vi "UpdateTimeout.vi"(7 "ReadOnlyIn":T1={"Qref"={"ValveCTR"=refnum, "Error"=refnum}, "UI_EN"=FALSE, "UserEventREF"={"TimeBasedProducer"={"Reg"=refnum, "Ref"=refnum}, "TimeBasedTempRead"={"Reg"=refnum, "Ref"=refnum}}, "UI_REF"=variant, "Paths"={"Log_Dir"=path "", "TempLog"=path "", "WateringLog"=path "", "Error"=path "", "Settings_Dir"=path "", "CFG.ini"=path "", "Plant_Digital_OP"=path "", "TimeTable"=path "", "Consol_Dir"=path "", "Input"=path "", "Output"=path "", "Timeout"=path "", "TimeoutTable"=path "", "Ch_Stat"=path "", "Temp"=path ""}, "PI_REF"={"IO"=enum."Remote", "Interface"=enum."Serial", "LINX Device Config"={"Interface"=enum."Serial", "COM Port"="COM13", "TCP Configuration"={"IP Address"="", "Port"=0}, "Device Family"=1, "Device ID"=1, "Device Name"="myRIO-1900", "TCP Ref"=refnum, "Channels"={"DI"=[0, 1, 2, 3, 4, 5, 6, 7, 8, 9, 10, 11, 12, 13, 14, 15, 16, 17, 18, 19, 20, 21, 22, 23, 24, 25, 26, 27, 28, 29, 30, 31, 32, 33, 34, 35, 36, 37, 38, 39, 40, 41, 42, 43, 44, 45, 46], "DO"=[0, 1, 2, 3, 4, 5, 6, 7, 8, 9, 10, 11, 12, 13, 14, 15, 16, 17, 18, 19, 20, 21, 22, 23, 24, 25, 26, 27, 28, 29, 30, 31, 32, 33, 34, 35, 36, 37, 38, 39, 40, 41, 42, 43, 44, 45, 46], "AI"=[0, 1, 2, 3, 4, 5, 6, 7, 8, 9, 10, 11], "AO"=[], "PWM"=[3, 5, 6, 9, 10], "QE"=[], "UART"=[0, 1], "I2C 2"=[0], "SPI"=[0], "CAN"=[], "Servo"=[], "AI Ref (V)"=0.0, "AI Resolution (Bits)"=0, "AO Ref (V)"=0.0, "AO Resolution (Bits)"=0}}}, "CFG"={"ProducerEn_PC"=FALSE, "Producer_PC_ms"=0, "ProducerEn_PI"=FALSE, "Producer_PI_ms"=0, "TempLogInterval"=15, "SystemResetTime"=0.0}} {"CFG"."SystemResetTime" format="%<%H:%M:%S>t"}, 8 "Error In":errorcluster, 11 "Read_WriteIN":T9={"Time Table"=[{"Set Time"=0.0, "Control"=enum."Time", "Duration[S]"=3.0, "Liter"=0.0, "Plant Name."="", "Watered"=FALSE, "Su"=FALSE, "Mo"=FALSE, "Tu"=FALSE, "We"=FALSE, "Th"=FALSE, "Fr"=FALSE, "Sa"=FALSE}, {"Set Time"=0.0, "Control"=enum."Time", "Duration[S]"=5.0, "Liter"=0.0, "Plant Name."="", "Watered"=FALSE, "Su"=FALSE, "Mo"=FALSE, "Tu"=FALSE, "We"=FALSE, "Th"=FALSE, "Fr"=FALSE, "Sa"=FALSE}, {"Set Time"=0.0, "Control"=enum."Time", "Duration[S]"=5.0, "Liter"=0.0, "Plant Name."="", "Watered"=FALSE, "Su"=FALSE, "Mo"=FALSE, "Tu"=FALSE, "We"=FALSE, "Th"=FALSE, "Fr"=FALSE, "Sa"=FALSE}], "Plants_Digital_OP"=[], "delta_ms_w_Index"={"delta_ms"=[], "Index"=[], "RunArray"=[]}, "TimeOutInfo"={"Timeout"=0, "ValveCTR"={"State"=enum."Open Valve", "Channel No"=0, "Duration[S]"=0.0}, "Index"=0}, "LoopName"=""} {"TimeOutInfo"."ValveCTR"."Channel No" items=["7"=7, "11"=11, "12"=12, "13"=13, "15"=15, "16"=16, "18"=18, "29"=29, "32"=32, "33"=33, "35"=35, "36"=36, "37"=37, "38"=38, "40"=40]; "delta_ms_w_Index"."RunArray"."Channel No" items=["7"=7, "11"=11, "12"=12, "13"=13, "15"=15, "16"=16, "18"=18, "29"=29, "32"=32, "33"=33, "35"=35, "36"=36, "37"=37, "38"=38, "40"=40]; "Plants_Digital_OP"."Channel No" items=["7"=7, "11"=11, "12"=12, "13"=13, "15"=15, "16"=16, "18"=18, "29"=29, "32"=32, "33"=33, "35"=35, "36"=36, "37"=37, "38"=38, "40"=40]; "Time Table"."Liter" min=0.0; "Time Table"."Set Time" format="%<%H:%M:%S>t"; "Time Table"."Duration[S]" min=0.0}) -> (0 "Error Out":errorcluster, 3 "Read_WriteOUT":T9={"Time Table"=[{"Set Time"=0.0, "Control"=enum."Time", "Duration[S]"=3.0, "Liter"=0.0, "Plant Name."="", "Watered"=FALSE, "Su"=FALSE, "Mo"=FALSE, "Tu"=FALSE, "We"=FALSE, "Th"=FALSE, "Fr"=FALSE, "Sa"=FALSE}, {"Set Time"=0.0, "Control"=enum."Time", "Duration[S]"=5.0, "Liter"=0.0, "Plant Name."="", "Watered"=FALSE, "Su"=FALSE, "Mo"=FALSE, "Tu"=FALSE, "We"=FALSE, "Th"=FALSE, "Fr"=FALSE, "Sa"=FALSE}, {"Set Time"=0.0, "Control"=enum."Time", "Duration[S]"=5.0, "Liter"=0.0, "Plant Name."="", "Watered"=FALSE, "Su"=FALSE, "Mo"=FALSE, "Tu"=FALSE, "We"=FALSE, "Th"=FALSE, "Fr"=FALSE, "Sa"=FALSE}], "Plants_Digital_OP"=[], "delta_ms_w_Index"={"delta_ms"=[], "Index"=[], "RunArray"=[]}, "TimeOutInfo"={"Timeout"=0, "ValveCTR"={"State"=enum."Open Valve", "Channel No"=0, "Duration[S]"=0.0}, "Index"=0}, "LoopName"=""} {"TimeOutInfo"."ValveCTR"."Channel No" items=["7"=7, "11"=11, "12"=12, "13"=13, "15"=15, "16"=16, "18"=18, "29"=29, "32"=32, "33"=33, "35"=35, "36"=36, "37"=37, "38"=38, "40"=40]; "delta_ms_w_Index"."RunArray"."Channel No" items=["7"=7, "11"=11, "12"=12, "13"=13, "15"=15, "16"=16, "18"=18, "29"=29, "32"=32, "33"=33, "35"=35, "36"=36, "37"=37, "38"=38, "40"=40]; "Plants_Digital_OP"."Channel No" items=["7"=7, "11"=11, "12"=12, "13"=13, "15"=15, "16"=16, "18"=18, "29"=29, "32"=32, "33"=33, "35"=35, "36"=36, "37"=37, "38"=38, "40"=40]; "Time Table"."Liter" min=0.0; "Time Table"."Set Time" format="%<%H:%M:%S>t"; "Time Table"."Duration[S]" min=0.0})   [LabVIEW 2020, in "TimeBasedProd.lvlib"]
uses:
  TimeBasedProd.lvlib
  TypeDef/Read_Write.ctl
  TimeTable/TypeDef/Time_Table.ctl
  TimeTable/TypeDef/Time_Table_CTR.ctl
  Digital_OP/TypeDef/Plant_OP_Map.ctl
  Digital_OP/TypeDef/Plant_OP_Map_CTR.ctl
  ValveCTRL/TypeDef/CHs_List.ctl
  TypeDef/TimeOutInfo.ctl
  ValveCTRL/TypeDef/Queue_Cluster.ctl
  ValveCTRL/TypeDef/States_Enum.ctl
  TypeDef/UpdateTimeOutinfo.ctl
  Main/TypeDef/ReadOnly.ctl
  Main/TypeDef/EventData.ctl
  <vilib>/MakerHub/LINX/Private/Type Defs/LINX Ref.ctl
  <vilib>/MakerHub/LINX/Private/Type Defs/Platform.ctl
  <vilib>/MakerHub/LINX/Private/Type Defs/Interface.ctl
  <vilib>/MakerHub/LINX/Private/Device/Type Defs/LINX Device Config.ctl
  <vilib>/MakerHub/LINX/Private/Device/Type Defs/TCP Config.ctl
  <vilib>/MakerHub/LINX/Private/Device/Type Defs/Channels.ctl
  Main/Init/ReadInitCFG/TypeDef/CFG_Cluster.ctl
  Time/Time.lvlib
  ValveCTRL/ValveCTRL.lvlib
  Main/Main.lvlib
  <vilib>/MakerHub/LINX/LMH-LINX.lvlib
  <vilib>/MakerHub/LINX/Private/Device/Device.lvlib
panel:
  # "Watering Days"
  # "Watering Days"
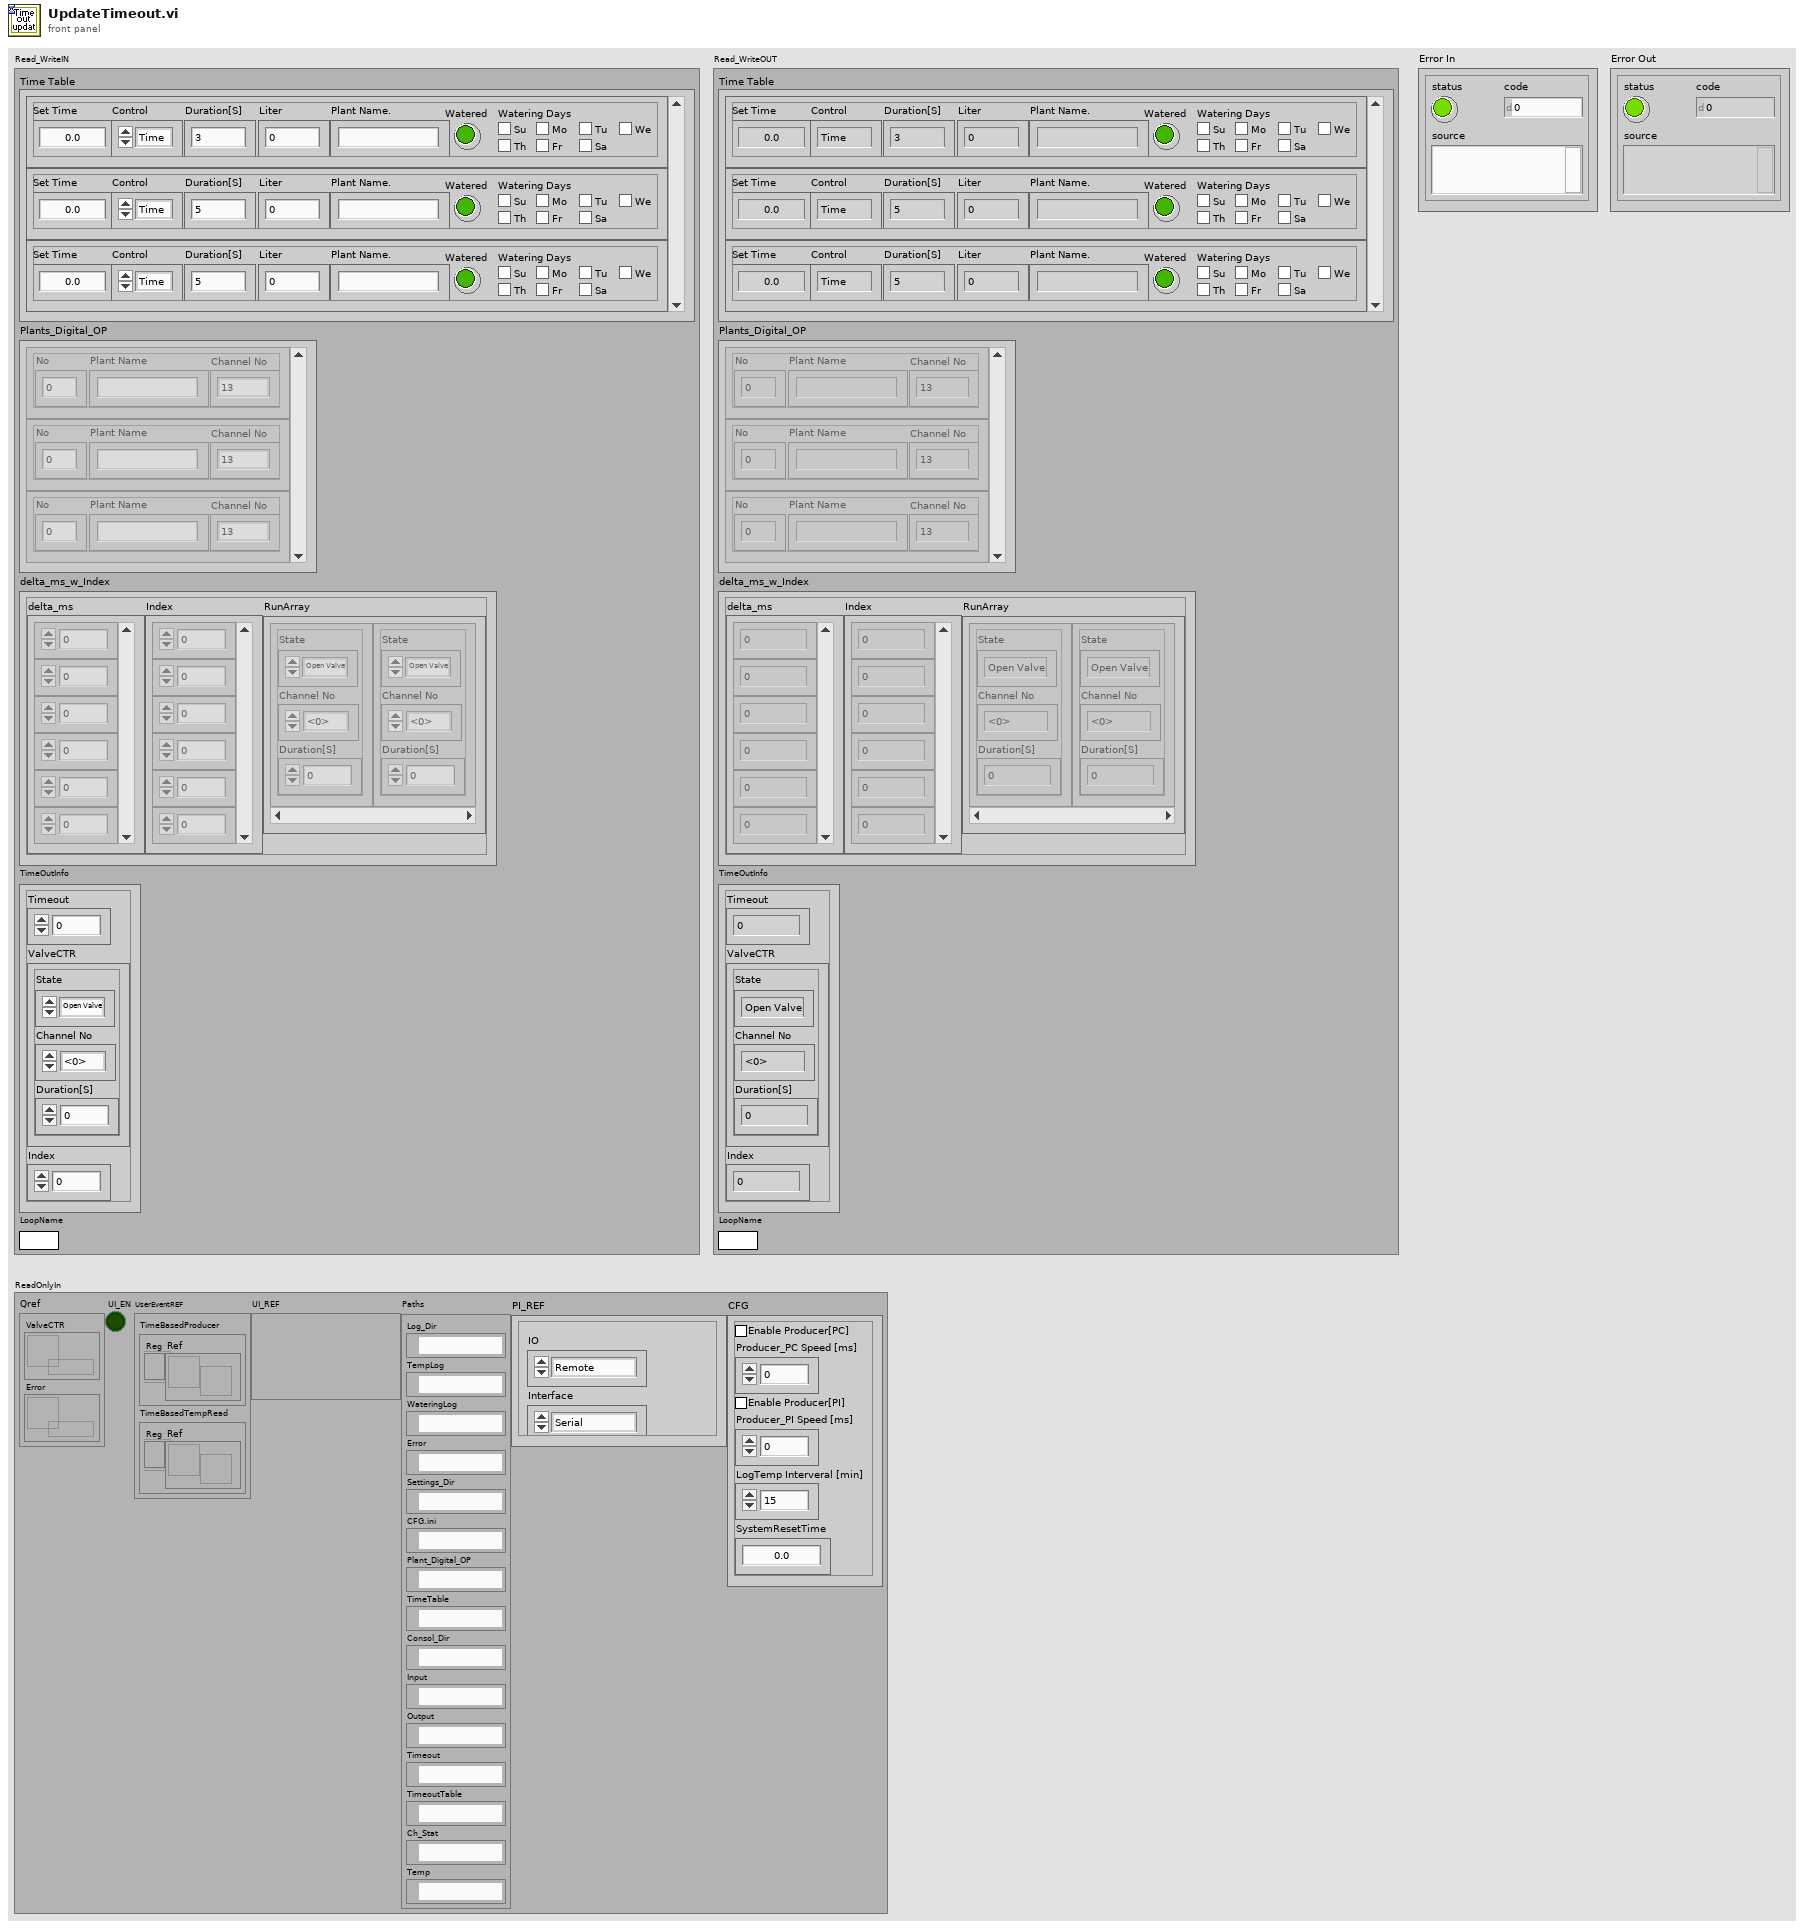
[diagram p1: front panel]
types:
  T1 = typedef "Main.lvlib/ReadOnly.ctl" = cluster{"Qref":cluster{"ValveCTR":refnum<queue>, "Error":refnum<queue>}, "UI_EN":bool, "UserEventREF":cluster{"TimeBasedProducer":cluster{"Reg":refnum<event-registration>, "Ref":refnum<user-event>}, "TimeBasedTempRead":cluster{"Reg":refnum<event-registration>, "Ref":refnum<user-event>}}, "UI_REF":variant, "Paths":cluster{"Log_Dir":path, "TempLog":path, "WateringLog":path, "Error":path, "Settings_Dir":path, "CFG.ini":path, "Plant_Digital_OP":path, "TimeTable":path, "Consol_Dir":path, "Input":path, "Output":path, "Timeout":path, "TimeoutTable":path, "Ch_Stat":path, "Temp":path}, "PI_REF":T2, "CFG":T8}
  T2 = typedef "LMH-LINX.lvlib/LINX Ref.ctl" = cluster{"IO":T3, "Interface":T4, "LINX Device Config":T5}
  T3 = typedef "LMH-LINX.lvlib/Platform.ctl" = enum16{"Remote", "Local"}
  T4 = typedef "LMH-LINX.lvlib/Interface.ctl" = enum16{"Serial", "TCP"}
  T5 = typedef "LMH-LINX.lvlib/Device.lvlib/LINX Device Config.ctl" = cluster{"Interface":T4, "COM Port":refnum<visa-resource-name>, "TCP Configuration":T6, "Device Family":u8, "Device ID":u8, "Device Name":string, "TCP Ref":refnum<k5>, "Channels":T7}
  T6 = typedef "LMH-LINX.lvlib/Device.lvlib/TCP Config.ctl" = cluster{"IP Address":string, "Port":u16}
  T7 = typedef "LMH-LINX.lvlib/Channels.ctl" = cluster{"DI":u8[], "DO":u8[], "AI":u8[], "AO":u8[], "PWM":u8[], "QE":u8[], "UART":u8[], "I2C 2":u8[], "SPI":u8[], "CAN":u8[], "Servo":u8[], "AI Ref (V)":dbl, "AI Resolution (Bits)":u8, "AO Ref (V)":dbl, "AO Resolution (Bits)":u8}
  T8 = typedef "Main.lvlib/CFG_Cluster.ctl" = cluster{"ProducerEn_PC":bool, "Producer_PC_ms":u32, "ProducerEn_PI":bool, "Producer_PI_ms":u32, "TempLogInterval":u32, "SystemResetTime":dbl}
  T9 = typedef "TimeBasedProd.lvlib/Read_Write.ctl" = cluster{"Time Table":T10, "Plants_Digital_OP":T12, "delta_ms_w_Index":T15, "TimeOutInfo":T18, "LoopName":string}
  T10 = typedef "TimeBasedProd.lvlib/Time_Table.ctl" = T11[]
  T11 = typedef "TimeBasedProd.lvlib/Time_Table_CTR.ctl" = cluster{"Set Time":dbl, "Control":enum16{"Time", "Flow"}, "Duration[S]":dbl, "Liter":dbl, "Plant Name.":string, "Watered":bool, "Su":bool, "Mo":bool, "Tu":bool, "We":bool, "Th":bool, "Fr":bool, "Sa":bool}
  T12 = typedef "TimeBasedProd.lvlib/Plant_OP_Map.ctl" = T13[]
  T13 = typedef "TimeBasedProd.lvlib/Plant_OP_Map_CTR.ctl" = cluster{"No":u8, "Plant Name":string, "Channel No":T14}
  T14 = typedef "ValveCTRL.lvlib/CHs_List.ctl" = u8
  T15 = typedef "TimeBasedProd.lvlib/TimeOutInfo.ctl" = cluster{"delta_ms":i32[], "Index":i32[], "RunArray":T16[]}
  T16 = typedef "ValveCTRL.lvlib/Queue_Cluster.ctl" = cluster{"State":T17, "Channel No":T14, "Duration[S]":dbl}
  T17 = typedef "ValveCTRL.lvlib/States_Enum.ctl" = enum16{"Open Pump", "Open Valve", "Wait Valve", "Close Pump", "Close Valve", "Save State", "StopLoop", "ValidCh"}
  T18 = typedef "TimeBasedProd.lvlib/UpdateTimeOutinfo.ctl" = cluster{"Timeout":i32, "ValveCTR":T16, "Index":i32}
  T19 = enum16{"open", "replace", "create", "open or create", "replace or create", "replace or create with confirmation"}
  T20 = typedef "Time.lvlib/Local_DateTime_String.ctl" = cluster{"Local Date Time":string, "Local Date":string, "Local Time":string}
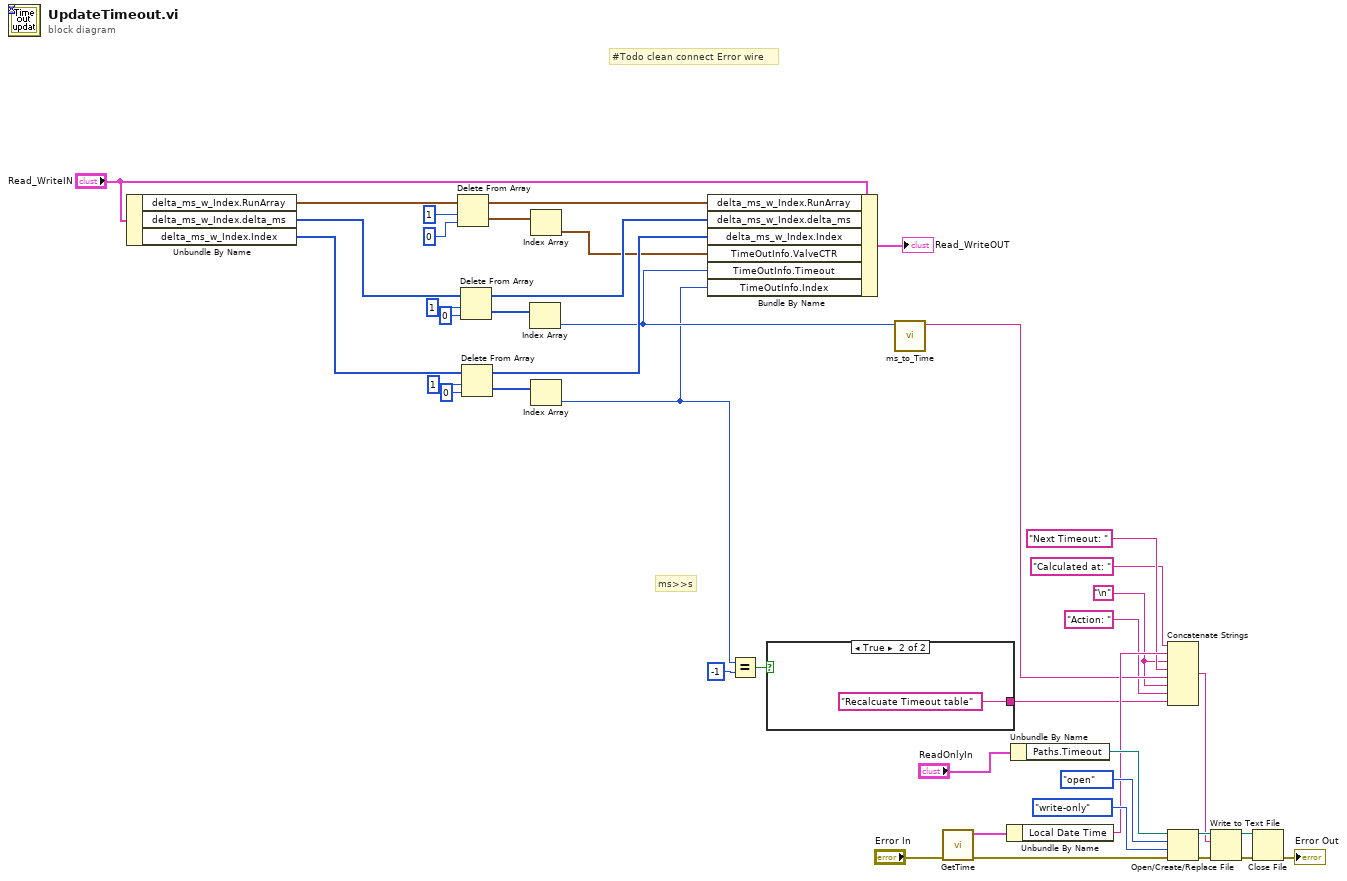
[diagram p0: block diagram]
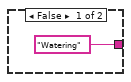
[diagram p2: hidden frame]
diagram:
  w3 = "\n"
  # "ms>>s"
  # "#Todo clean connect Error wire"
  n1 = Unbundle By Name("Read_WriteIN") -> ("delta_ms_w_Index.RunArray"=w33:T16[], "delta_ms_w_Index.delta_ms"=w41:i32[], "delta_ms_w_Index.Index"=w29:i32[])
  n2 = Delete From Array(array=w33, length=1, index=0) -> (deleted portion=w40:T16[], array with subset deleted=w34:T16[])
  n3 = Delete From Array(array=w41, length=1, index=0) -> (deleted portion=w37:i32[], array with subset deleted=w42:i32[])
  n4 = Delete From Array(array=w29, length=1, index=0) -> (deleted portion=w32:i32[], array with subset deleted=w28:i32[])
  n5 = Index Array(array=w37) -> (element=w8:i32)  [unwired: 1 in]
  n6 = Index Array(array=w40) -> (element=w26:T16)  [unwired: 1 in]
  n7 = Index Array(array=w32) -> (element=w6:i32)  [unwired: 1 in]
  n8 = Bundle By Name(cluster="Read_WriteIN", "delta_ms_w_Index.RunArray"=w34, "delta_ms_w_Index.delta_ms"=w42, "delta_ms_w_Index.Index"=w28, "TimeOutInfo.ValveCTR"=w26, "TimeOutInfo.Timeout"=w8, "TimeOutInfo.Index"=w6) -> (→"Read_WriteOUT":T9)
  n9 = Equal?(x=w6, y=-1) -> (x = y?=w4:bool)
  n10 = case shown="True" w4 {
    tunnel: ["Watering" ("string") "Recalcuate Timeout table" ("string")] -> w1
    frame False {
    }
    frame True {
    }
  }
  n11 = call "ms_to_Time.vi"("TimeOut[ms]"=w8) -> ("Time[String]"=w16:string)  [unwired: 10 in]
  n12 = call "GetTime.vi"("error in"="Error In") -> ("error out"=w10:errorcluster, "Local Data/Time[String]"=w18:T20)  [unwired: 8 in, 1 out]
  n13 = Unbundle By Name(w18) -> ("Local Date Time"=w17:string)
  n14 = Unbundle By Name("ReadOnlyIn") -> ("Paths.Timeout"=w23:path)
  n15 = Concatenate Strings("Calculated at: " ("string"), w17, w3, "Next Timeout: " ("string"), w16, w3, "Action: " ("string"), w1) -> (w14:string)
  n16 = Open/Create/Replace File(file path (use dialog)=w23, error in=w10, operation (0:open)=T19."open", access (0:read/write)=enum16{"read/write", "read-only", "write-only"}."write-only") -> (refnum out=w19:refnum<file>, error out=w20:errorcluster)  [unwired: 2 in, 1 out]
  n17 = Write to Text File(file (use dialog)=w19, text=w14, error in=w20) -> (refnum out=w12:refnum<file>, error out=w13:errorcluster)  [unwired: 1 in, 1 out]
  n18 = Close File(refnum=w12, error in=w13) -> (error out=→"Error Out":errorcluster)  [unwired: 1 out]
